vi "Memory.Array.Dispose.vi"(8 "error in (no error)":errorcluster, 11 "Array in":refnum<class "Memory.Array.Void.lvclass">) -> (0 "error out":errorcluster)   [LabVIEW 2016, in "LabVIEW Memory Manager.lvlib" / "Memory.Array.Void.lvclass"]
uses:
  Memory.Array.Void.lvclass
  Memory.Array.Void.lvclass/Memory.Array.Void.ctl
  Pointer/Pointer.Void/Memory.Pointer.Void.lvclass/Memory.Pointer.Void.ctl
  Pointer/Pointer.Void/Methods/Memory.Pointer.Get Address.vi
  Pointer/Pointer.Void/Memory.Pointer.Void.lvclass
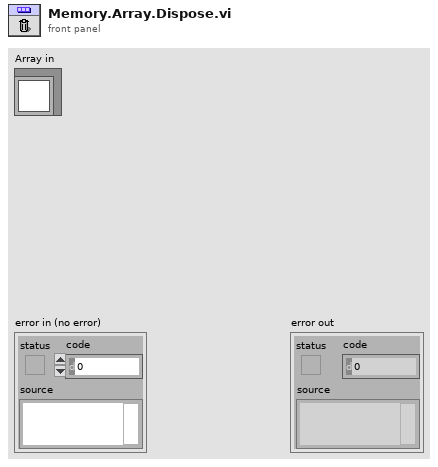
[diagram p1: front panel]
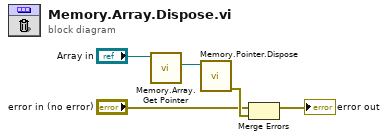
[diagram p0: block diagram]
diagram:
  n1 = call "Memory.Array.Get Pointer.vi"("Array in"="Array in") -> ("Pointer"=w5:refnum<class "Memory.Pointer.Void.lvclass">)  [unwired: 8 in, 2 out]
  n2 = call "Memory.Pointer.Dispose.vi"("Pointer in"=w5) -> ("error out"=w4:errorcluster)  [unwired: 10 in]
  n3 = Merge Errors("error in (no error)", w4) -> (→"error out":errorcluster)
